vi "Example Digital.vi"() -> ()   [LabVIEW 2015]
uses:
  Controls/SampleRateControlDig.ctl
  <vilib>/Waveform/DWDTOps.llb/Digital Pattern Generator (Ramp).vi
  <vilib>/Waveform/DWDTOps.llb/DWDT Digital to Binary U32.vi
panel:
  in  "Stop and Disconnect":bool
  in  "Samples / chn IN":i32=8192
  out "Digital\nWaveform\nGraph 2":digitalwaveform(graph)
  in  "Samplerate In":T1=8192 min=10 max=100000000 step=10
  in  "Samplerate Out":T1=8192 caption="Samplerate In" min=10 max=100000000 step=10
  in  "Samples / chn out":u32=8192
  in  "Active ADALM2000 URIs:":u16(ring) items=["ip:192.168.2.1", "usb:1.6.5", "usb:1.6.5"]
  in  "Connect Btn":bool
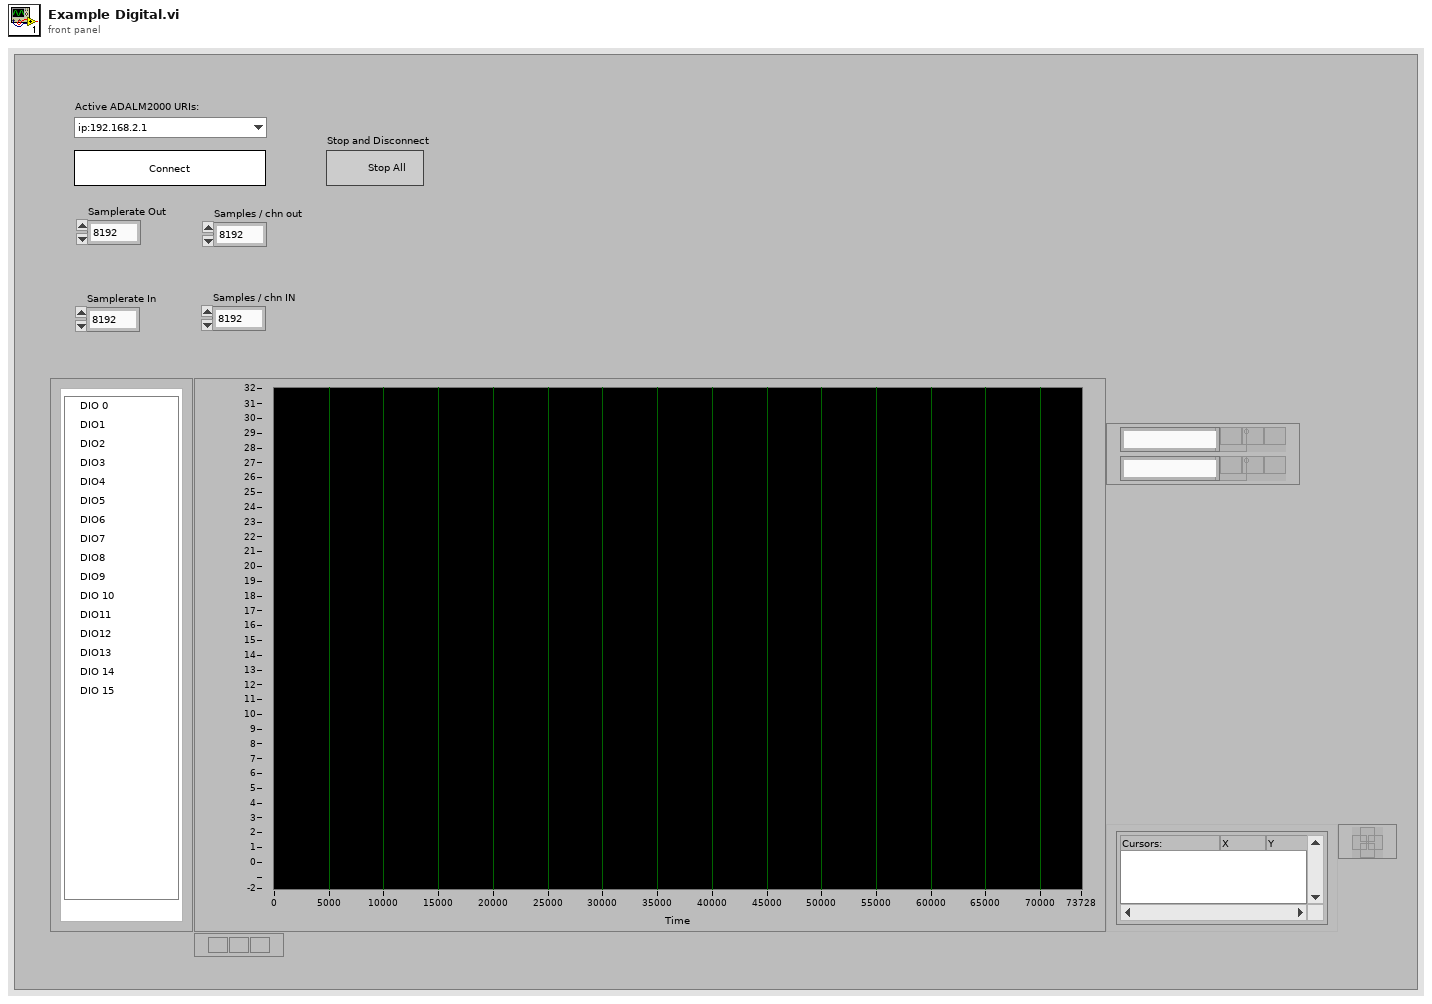
[diagram p1: front panel]
types:
  T1 = typedef "SampleRateControlDig.ctl" = i32
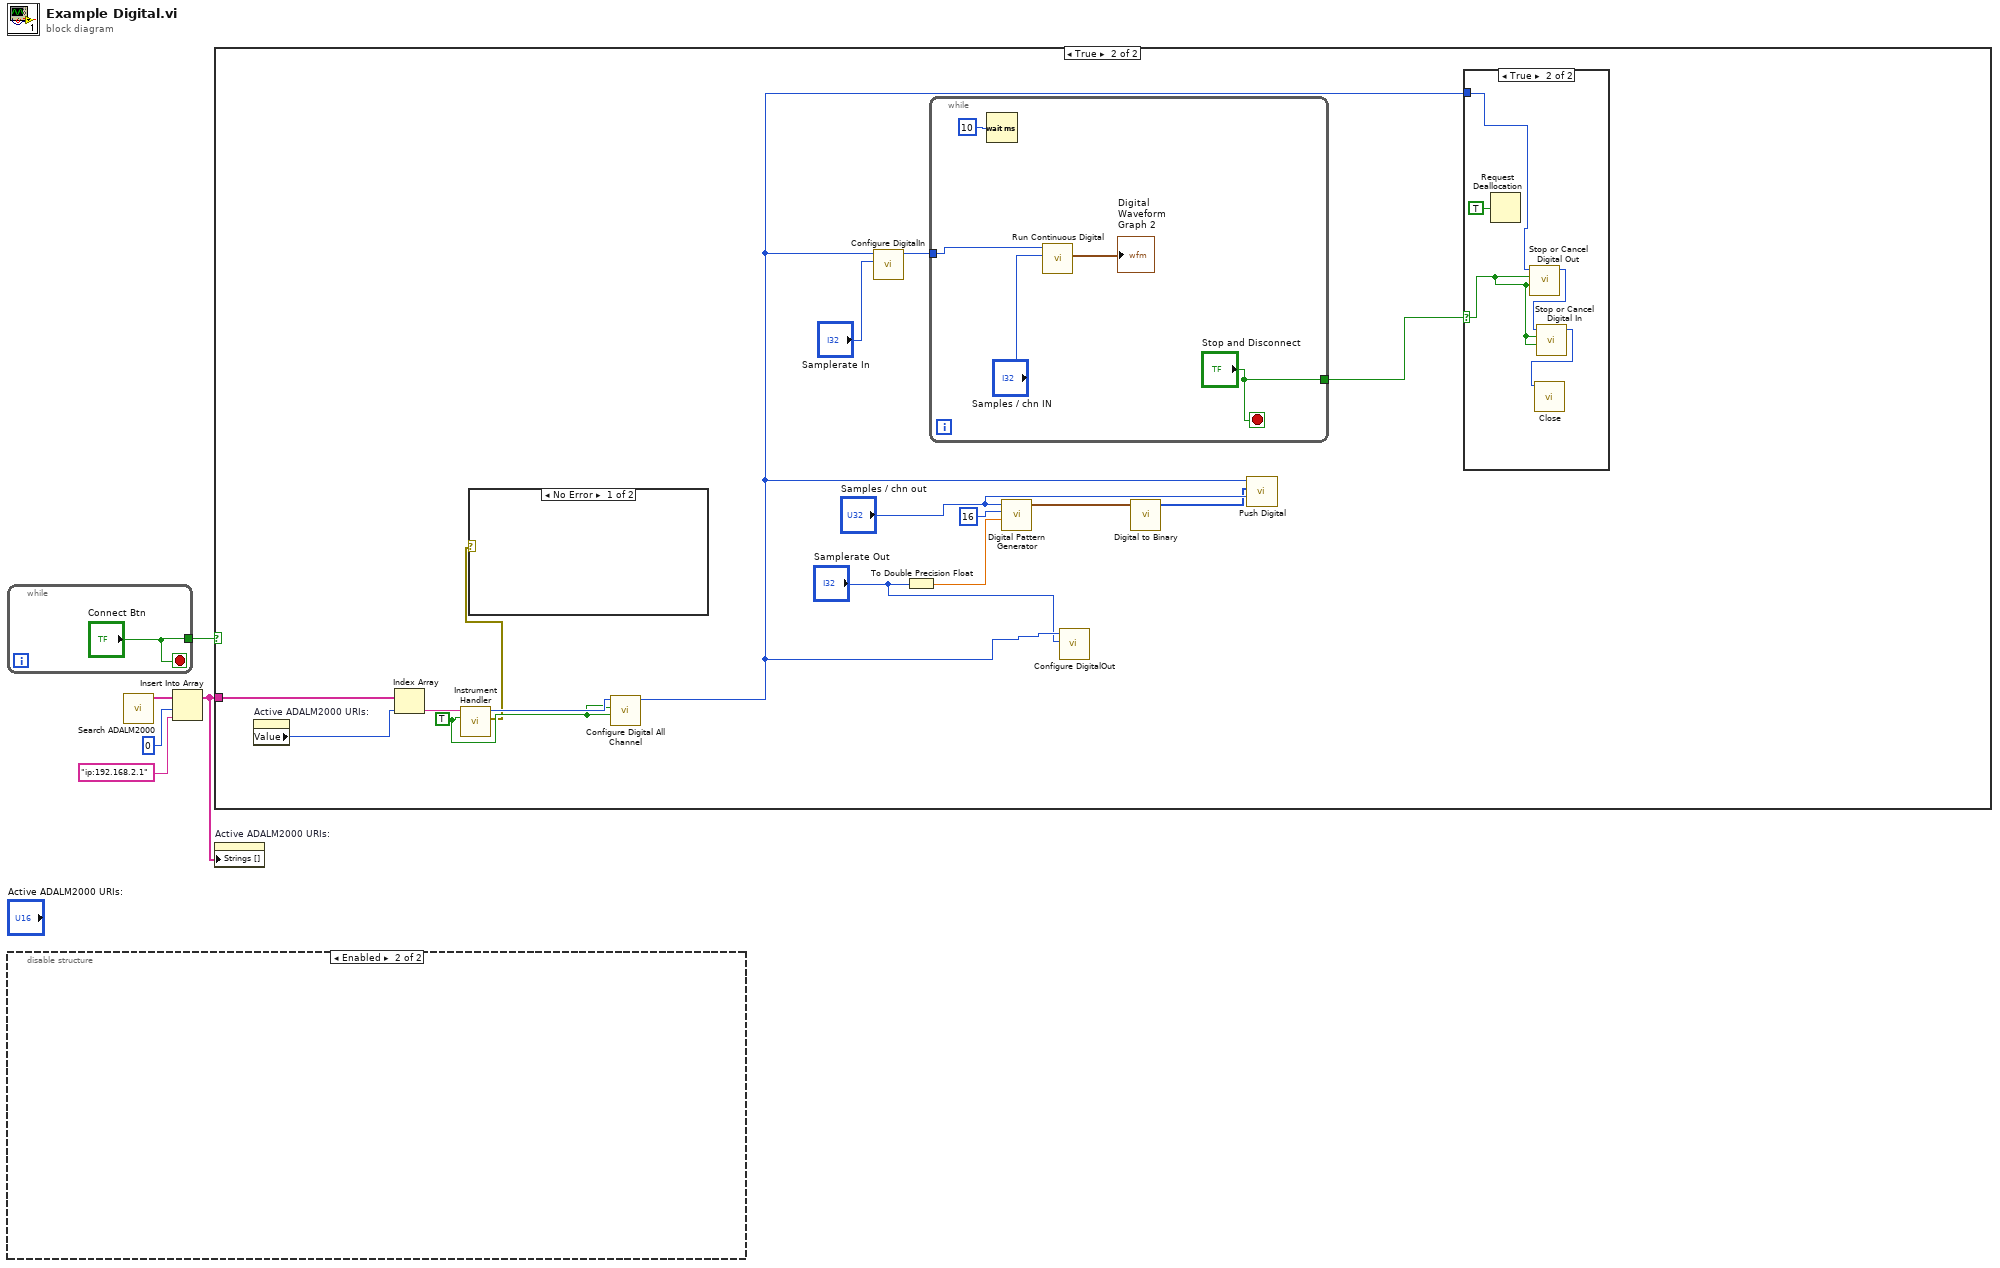
[diagram p0: block diagram]
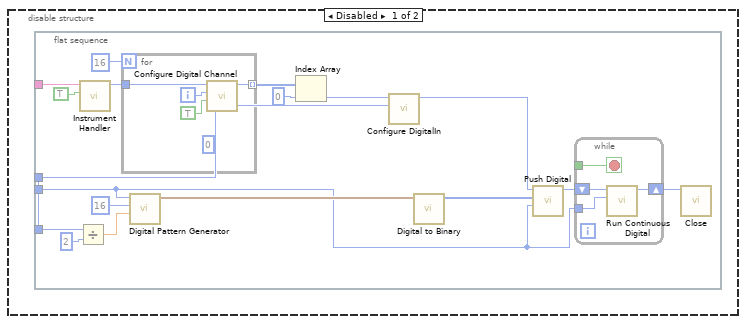
[diagram p2: hidden frame]
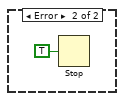
[diagram p4: hidden frame]
diagram:
  n1 = while {
    tunnel: ["Connect Btn"] -> w1
    stop <- "Connect Btn" stop-if-true
  }
  n2 = disable-structure shown="Enabled" {
    frame Disabled {
      n3 = flat-sequence {
        tunnel: [w21] -> w9
        tunnel: [w14] -> w8
        tunnel: [w19] -> w7
        tunnel: w7 -> [w13]
        frame #0 {
          n4 = Divide(x=w13, y=T1 2) -> (x/y=w11:dbl)
          n5 = call "Instrument Handler.vi"("Calibrate"=TRUE, "ADALM2000 URI"=w21) -> ("ADALM2000 Handle"=w26:u32)  [unwired: 8 in, 1 out]
          n6 = for {
            N: 16 -> [_]
            tunnel: w26 -> [w36]
            tunnel: [w35] -> w24 mode=indexing
            i -> [w34]
            (unwired) 0
            n7 = call "Configure Digital Channel.vi"("Output"=TRUE ("Enable"), "channel"=w34, "ADALM2000 In"=w36) -> ("ADALM2000 Out"=w35:u32)  [unwired: 8 in]
          }
          n8 = call-poly <vilib>:"Digital Pattern Generator.vi"("sample rate"=w11, "number of signals"=u32 16, "number of samples"=w14) -> ("digital waveform"=w18:digitalwaveform)  [unwired: 7 in, 1 out]
          n9 = Index Array(array=w24, index=0) -> (element=w20:u32)
          n10 = call "Configure DigitalIn.vi"("Samplerate In"=w19, "ADALM2000 Handler"=w20) -> ("ADALM2000 Handler 2"=w16:u32)  [unwired: 9 in]
          n11 = call-poly <vilib>:"Digital to Binary.vi"("digital waveform"=w18) -> ("binary array"=w17:u32[])  [unwired: 9 in, 1 out]
          n12 = call "Push Digital.vi"("Sample count"=w14, "digital_samples"=w17, "ADALM2000 Handler"=w16) -> ("ADALM2000 Handler 2"=w15:u32)  [unwired: 8 in]
          n13 = while {
            shift-right: [w30] -> w22
            shift-left: w15 -> [w31]
            tunnel: _ -> [w32]
            tunnel: w14 -> [w29]
            stop <- w32 stop-if-true
            n14 = call "Run Continuous Digital.vi"("Samples / channel"=w29, "ADALM2000 Handler"=w31) -> ("output waveform"=w28:digitalwaveform, "ADALM2000 Handler 2"=w30:u32)  [unwired: 7 in]
          }
          n15 = call "Close.vi"("ADALM2000 Handler"=w22) -> ()  [unwired: 11 in]
        }
      }
    }
    frame Enabled {
    }
  }
  n16 = call "Search ADALM2000.vi"() -> ("Array"=w5:string[])  [unwired: 11 in]
  n17 = Insert Into Array(array=w5, index=0, new element="ip:192.168.2.1" ("new element/subarray")) -> (w2:string[])
  n18 = case shown="True" w1 {
    tunnel: w2 -> [_ w50]
    frame False {
    }
    frame True {
      w48 = TRUE ("Calibrate")
      n19 = property on="Active ADALM2000 URIs:" class="Ring (strict)"() -> ("Value"=w52:u16)  [unwired: 2 in, 2 out]
      n20 = Index Array(array=w50, index=w52) -> (element=w51:string)
      n21 = call "Instrument Handler.vi"("Calibrate"=w48, "ADALM2000 URI"=w51) -> ("error out"=w47:errorcluster, "ADALM2000 Handle"=w49:u32)  [unwired: 8 in]
      n22 = case shown="No Error" w47 {
        frame No Error {
        }
        frame Error {
          n23 = Stop(stop? (T)=TRUE) -> ()
        }
      }
      n24 = call "Configure Digital All Channel.vi"("Cyclic"=w48, "Output"=w48, "ADALM2000 In"=w49) -> ("ADALM2000 Out"=w38:u32)  [unwired: 8 in]
      n25 = call "Configure DigitalIn.vi"("Samplerate In"="Samplerate In", "ADALM2000 Handler"=w38) -> ("ADALM2000 Handler 2"=w40:u32)  [unwired: 9 in]
      n26 = To Double Precision Float(number="Samplerate Out") -> (double precision float=w43:dbl)
      n27 = while {
        tunnel: w40 -> [w60]
        tunnel: ["Stop and Disconnect"] -> w39
        stop <- "Stop and Disconnect" stop-if-true
        n28 = Wait (ms)(milliseconds to wait=u32 10) -> ()  [unwired: 1 out]
        n29 = call "Run Continuous Digital.vi"("Samples / channel"="Samples / chn IN", "ADALM2000 Handler"=w60) -> ("output waveform"=→"Digital\nWaveform\nGraph 2":digitalwaveform)  [unwired: 7 in, 1 out]
      }
      n30 = call-poly <vilib>:"Digital Pattern Generator.vi"("sample rate"=w43, "number of signals"=u32 16, "number of samples"="Samples / chn out") -> ("digital waveform"=w46:digitalwaveform)  [unwired: 7 in, 1 out]
      n31 = call "Configure DigitalOut.vi"("Samplerate Out"="Samplerate Out", "ADALM2000 Handler"=w38) -> ()  [unwired: 9 in, 1 out]
      n32 = call-poly <vilib>:"Digital to Binary.vi"("digital waveform"=w46) -> ("binary array"=w42:u32[])  [unwired: 9 in, 1 out]
      n33 = call "Push Digital.vi"("Sample count"="Samples / chn out", "digital_samples"=w42, "ADALM2000 Handler"=w38) -> ()  [unwired: 8 in, 1 out]
      n34 = case shown="True" w39 {
        selector: w39 -> [_ w55]
        tunnel: w38 -> [_ w57]
        frame False {
        }
        frame True {
          n35 = Request Deallocation(TRUE ("flag")) -> ()
          n36 = call "Stop or Cancel Digital Out.vi"("ADALM2000 Handler"=w57, "Cancel"=w55, "Stop"=w55) -> ("ADALM2000 Handler 2"=w56:u32)  [unwired: 7 in]
          n37 = call "Stop or Cancel Digital In.vi"("Stop"=w55, "Cancel"=w55, "ADALM2000 Handler"=w56) -> ("ADALM2000 Handler 2"=w54:u32)  [unwired: 8 in]
          n38 = call "Close.vi"("ADALM2000 Handler"=w54) -> ()  [unwired: 11 in]
        }
      }
    }
  }
  n39 = property on="Active ADALM2000 URIs:" class="Ring (strict)"("Strings []"=w2) -> ()  [unwired: 2 in, 2 out]
